vi "Target ID Map.vi"(8 "error in (no error)":errorcluster, 11 "Cluster in":refnum<class "Cluster.lvclass">) -> (0 "error out":errorcluster, 2 "Target ID Map":map{string, u32}(c390), 3 "Cluster out":refnum<class "Cluster.lvclass">)   [LabVIEW 2020, in "VolatusConfig.lvlib" / "Cluster.lvclass"]
uses:
  Cluster.lvclass
  C:/dev/lv20CE/relink/lv-volatus/VolatusConfig/VolatusConfigElement/VolatusConfigElement.lvclass
  Meta Type.ctl
  VolatusConfigElement/VolatusConfigElement.lvclass/VolatusConfigElement.ctl
  VolatusConfigElement/Element.vi
  Node/Node.lvclass
  lv-cdm/CDM-Config/Config Lookup/Match Meta.vi
  lv-cdm/CDM-Config/Config Element/Owner.vi
  lv-cdm/CDM-Config/Config Manager/Lookup Descendant.vi
  lv-cdm/CDM-Config/Config Filter/Config Lookup.lvclass
  Cluster.lvclass/Cluster.ctl
  VolatusConfigElement/VolatusConfigElement.lvclass
  VolatusConfig.lvlib
  C:/dev/lv20CE/relink/lv-volatus/VolatusConfig/Cluster/Cluster.lvclass
  lv-cdm/CDM-Config/Config Element/Config Element.lvclass
  C:/dev/lv20CE/relink/lv-volatus/VolatusConfig/Node/Node.lvclass
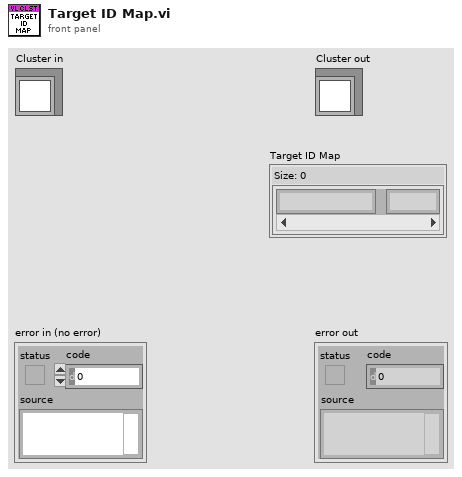
[diagram p1: front panel]
types:
  T1 = typedef "VolatusConfig.lvlib/Meta Type.ctl" = enum16{"UNKNOWN", "VL_System", "VL_Cluster", "VL_Node", "VL_Task", "VL_Group", "VL_Channel", "VL_Task_List", "VL_Scaling", "VL_Sensor", "VL_Sensor_List", "VL_Scale"}
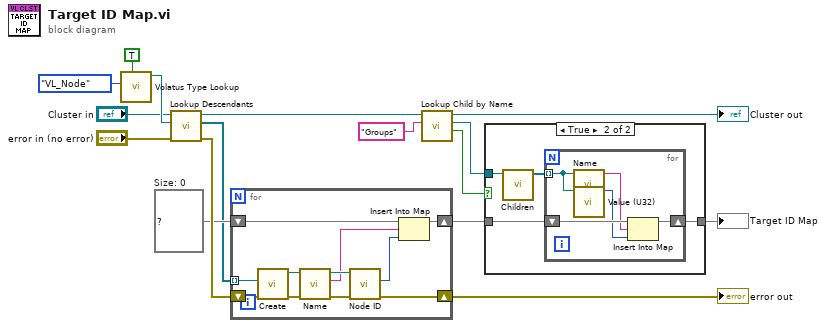
[diagram p0: block diagram]
diagram:
  w12 = map{string, u32} {}  # Size: 0
  n1 = call "Volatus Type Lookup.vi"("Don't Recurse Past Match (F)"=TRUE, "Meta Type"=Meta_Type."VL_Node") -> ("Config Lookup out"=w14:refnum<class "Config Lookup.lvclass">)  [unwired: 8 in, 1 out]
  n2 = call "Lookup Descendants.vi"("error in (no error)"="error in (no error)", "Lookup"=w14, "VolatusConfigElement in"="Cluster in") -> ("error out"=w16:errorcluster, "Descendants"=w11:refnum<class "Config Element.lvclass">[], "VolatusConfigElement out"=w8:refnum<class "Cluster.lvclass">)  [unwired: 6 in]
  n3 = for {
    shift-right: [w17] -> w3
    shift-left: w12 -> [w21]
    tunnel: w11 -> [w27] mode=indexing
    shift-right: [w18] -> w7
    shift-left: w16 -> [w25]
    n4 = call "Create.vi"("error in (no error)"=w25, "Element"=w27) -> ("error out"=w24:errorcluster, "Node out"=w26:refnum<class "Node.lvclass">)  [unwired: 8 in]
    n5 = call "Name.vi"("error in (no error)"=w24, "VolatusConfigElement in"=w26) -> ("error out"=w22:errorcluster, "Name"=w19:string, "VolatusConfigElement out"=w23:refnum<class "Node.lvclass">)  [unwired: 7 in]
    n6 = call "Node ID.vi"("error in (no error)"=w22, "Node in"=w23) -> ("error out"=w18:errorcluster, "Node ID"=w20:u32)  [unwired: 7 in, 1 out]
    n7 = Insert Into Map(map in=w21, key=w19, value=w20) -> (map out=w17:map{string, u32})  [unwired: 2 out]
  }
  "error out" <- w7
  n8 = call "Lookup Child by Name.vi"("Child Name"="Groups", "VolatusConfigElement in"=w8) -> ("Found"=w4:bool, "Child"=w2:refnum<class "Config Element.lvclass">, "VolatusConfigElement out"=→"Cluster out":refnum<class "Cluster.lvclass">)  [unwired: 6 in, 1 out]
  n9 = case shown="True" w4 {
    tunnel: w3 -> [w28 w30]
    tunnel: w2 -> [_ w32]
    tunnel: [w28 w29] -> w1
    frame False {
      # "Specifying target groups is optional."
    }
    frame True {
      n10 = call "Children.vi"("Config Element in"=w32) -> ("Elements"=w31:refnum<class "Config Element.lvclass">[])  [unwired: 9 in, 1 out]
      n11 = for {
        tunnel: w31 -> [w37] mode=indexing
        shift-right: [w33] -> w29
        shift-left: w30 -> [w36]
        n12 = call "Name.vi"("Config Element in"=w37) -> ("Name"=w34:string)  [unwired: 9 in, 1 out]
        n13 = call "Value (U32).vi"("Config Element in"=w37) -> ("U32 Value"=w35:u32)  [unwired: 9 in, 1 out]
        n14 = Insert Into Map(map in=w36, key=w34, value=w35) -> (map out=w33:map{string, u32})  [unwired: 2 out]
      }
    }
  }
  "Target ID Map" <- w1
